vi "Configure Critical Levels.vi"() -> (0 "STOP ALL OUT":bool)   [LabVIEW 2016]
uses:
  Typedef/Data_ID.ctl
  <vilib>/Utility/file.llb/Write Delimited Spreadsheet (DBL).vi
  <vilib>/Utility/file.llb/Read Delimited Spreadsheet (DBL).vi
panel:
  out "Names":string[](array[string])
  in  "Data ID Nr":T1 items=["", "", "", "", "", "MCU ADRESS", "", "", "", "", "ACC X", "ACC Y", "ACC Z", "ACC LEN", "TIME HOURS", "TIME MINUTS", "TIME SECONDS", "XBEE TEMP", "INSIDE TEMP", "OUTSIDE TEMP", "POT111", "PIR SENSOR", "LIGHT SENSOR", "", "", "DOOR STAUS_1", "DOOR STAUS_1", "", "", "", "Empty", "Empty", "Empty", "", "", "", "", "", "", "", "", "", "", "", "", "", "", "", "", "", "", "", "", "", "", "", "", "", "", "", "", "Empty"]
  in  "Load Button":bool
  in  "STOP ALL":bool
  in  "Exit":bool
  in  "Save Button":bool
  out "appended array":dbl[][](array[numeric])
  in  "Max Value":dbl[](array[numeric])=[0.0, 0.0, 0.0, 0.0, 0.0, 0.0, 0.0, 0.0, 0.0, 0.0, 0.0, 0.0, 0.0, 0.0, 0.0, 0.0, 0.0, 0.0, 0.0, 0.0]
  in  "On/Off Sensing":bool[](array[boolean])
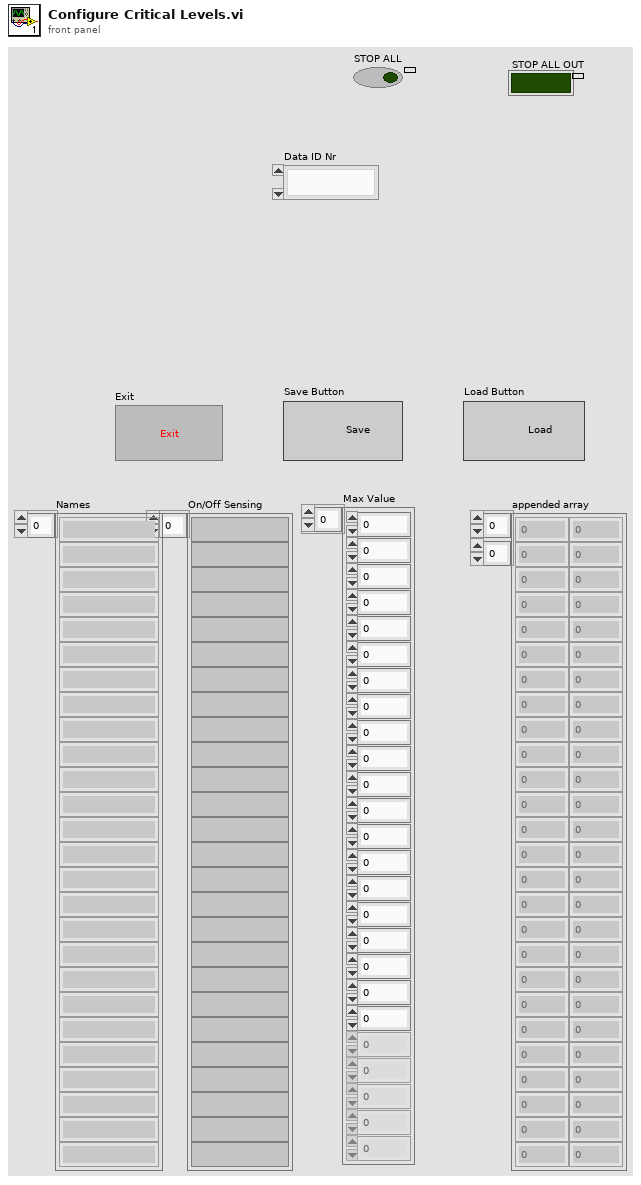
[diagram p1: front panel]
types:
  T1 = typedef "Data_ID.ctl" = u16
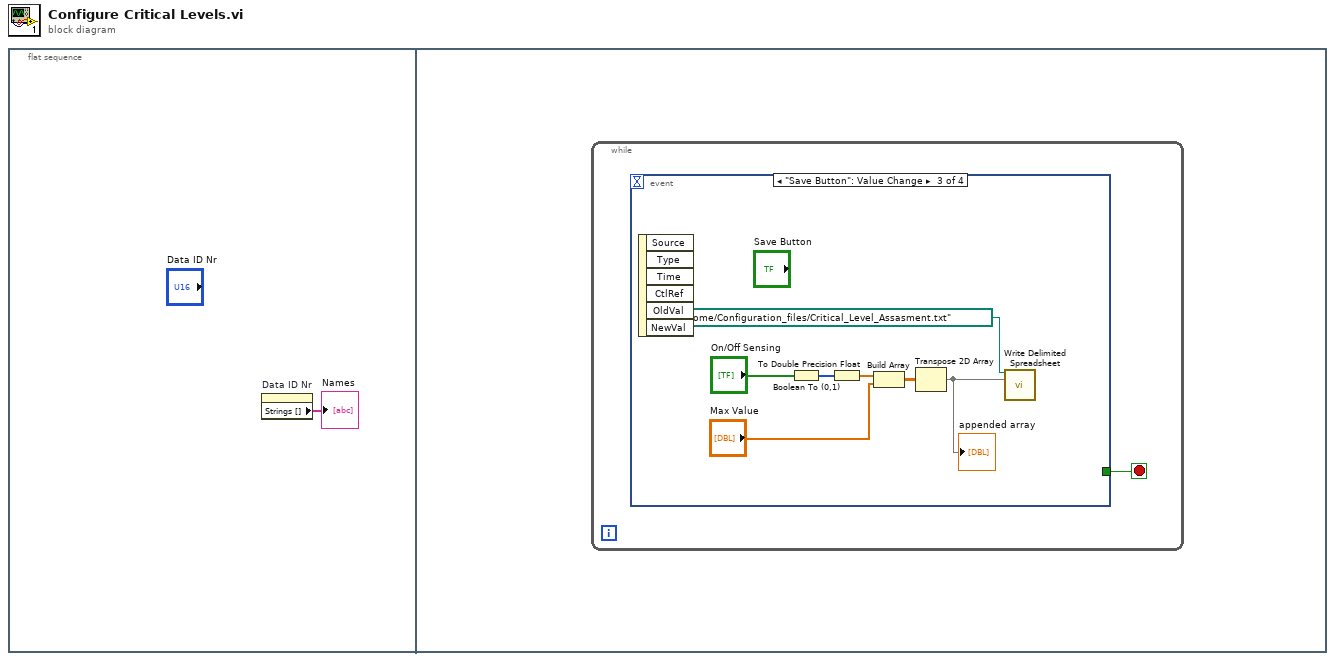
[diagram p0: block diagram]
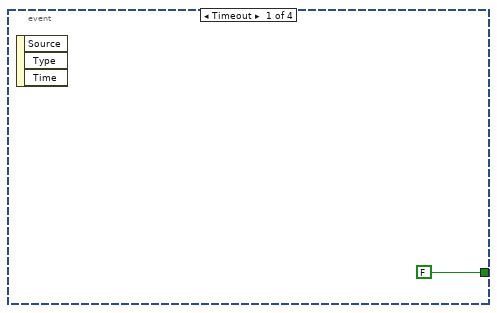
[diagram p2: hidden frame]
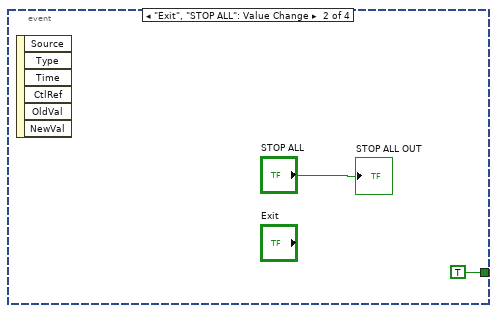
[diagram p3: hidden frame]
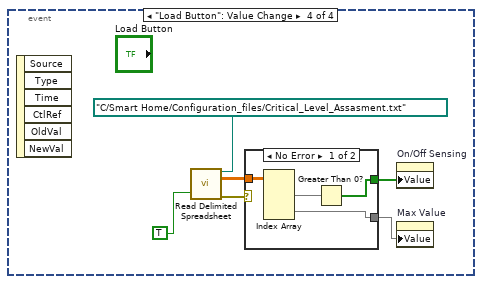
[diagram p4: hidden frame]
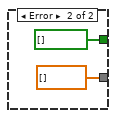
[diagram p5: hidden frame]
diagram:
  n1 = flat-sequence {
    frame #0 {
      n2 = property on="Data ID Nr" class="Ring (strict)"() -> ("Strings []"=→"Names":string[])  [unwired: 2 in, 2 out]
    }
    frame #1 {
      n3 = while {
        stop <- w2 stop-if-true
        n4 = event shown="[2] \"Save Button\": Value Change" {
          selector: _ -> [_ _ _ _]
          dyn-events: _ -> [_ _ _ _]
          timeout: _ -> [_ _ _ _]
          tunnel: [FALSE TRUE _ _] -> w2
          event Timeout {
            n5 = event-data() -> ()  [unwired: 1 in, 3 out]
          }
          event "Exit", "STOP ALL": Value Change {
            n6 = event-data() -> ()  [unwired: 1 in, 6 out]
            "STOP ALL OUT" <- "STOP ALL"
          }
          event "Save Button": Value Change {
            n7 = event-data() -> ()  [unwired: 1 in, 6 out]
            n8 = Boolean To (0,1)(Boolean="On/Off Sensing") -> (0, 1=w12:i16[])
            n9 = To Double Precision Float(number=w12) -> (double precision float=w8:dbl[])
            n10 = Build Array(w8, "Max Value") -> (w10:dbl[][])
            n11 = Transpose 2D Array(2D array=w10) -> (transposed array=w11:dbl[][])
            "appended array" <- w11
            n12 = call-poly <vilib>:"Write Delimited Spreadsheet.vi"("file path (dialog if empty)"=path "C:/Smart Home/Configuration_files/Critical_Level_Assasment.txt", "2D data"=w11) -> ()  [unwired: 12 in, 2 out]
          }
          event "Load Button": Value Change {
            n13 = event-data() -> ()  [unwired: 1 in, 6 out]
            n14 = call-poly <vilib>:"Read Delimited Spreadsheet.vi"("file path (dialog if empty)"=path "C:/Smart Home/Configuration_files/Critical_Level_Assasment.txt", "transpose? (F)"=TRUE) -> ("all rows"=w16:dbl[][], "error out"=w13:errorcluster)  [unwired: 8 in, 4 out]
            n15 = case shown="No Error" w13 {
              tunnel: [w19 dbl[] [] ("Min Values")] -> w14
              tunnel: [w22 bool[] []] -> w15
              tunnel: w16 -> [w21 _]
              frame No Error {
                n16 = Index Array(array=w21) -> (element #1=w20:dbl[], element #2=w19:dbl[])  [unwired: 4 in]
                n17 = Greater Than 0?(x=w20) -> (x > 0?=w22:bool[])
              }
              frame Error {
              }
            }
            n18 = property on="On/Off Sensing" class="Arr (strict)"("Value"=w15) -> ()  [unwired: 2 in, 2 out]
            n19 = property on="Max Value" class="Arr (strict)"("Value"=w14) -> ()  [unwired: 2 in, 2 out]
          }
        }
      }
    }
  }
